vi "VRM.Get Target.vi"(6 "Axis":T1=enum."Z", 8 "error in (no error)":errorcluster, 11 "Instrument.VRM in":refnum<class "Instrument.OxfordVRM.lvclass">) -> (0 "error out":errorcluster, 1 "Target Field Rate (T/min)":dbl[](array[numeric]), 2 "Target Field (T)":dbl[](array[numeric]), 3 "Instrument.VRM out":refnum<class "Instrument.OxfordVRM.lvclass">)   [LabVIEW 2019, in "Instrument.OxfordVRM.lvclass"]
uses:
  Instrument.OxfordVRM.lvclass
  Typedefs/VRM Magnet Axis--Enum.ctl
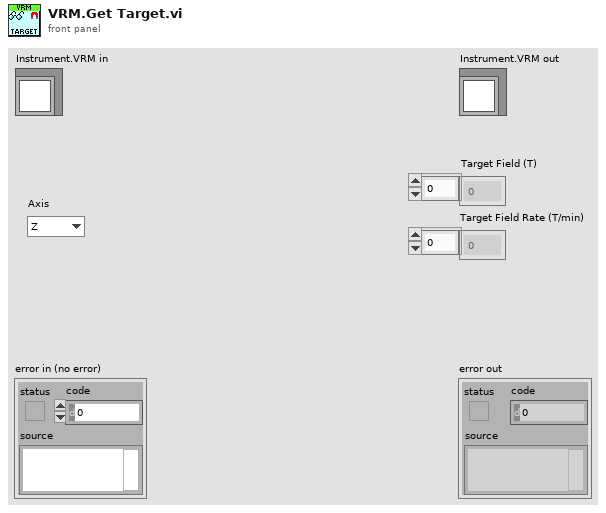
[diagram p1: front panel]
types:
  T1 = typedef "Instrument.OxfordVRM.lvclass/VRM Magnet Axis--Enum.ctl" = enum16{"X", "Y", "Z", "ALL"}
  T2 = typedef "Instrument.Cryostat.lvclass/Magnet Axis--Enum.ctl" = enum16{"X", "Y", "Z"}
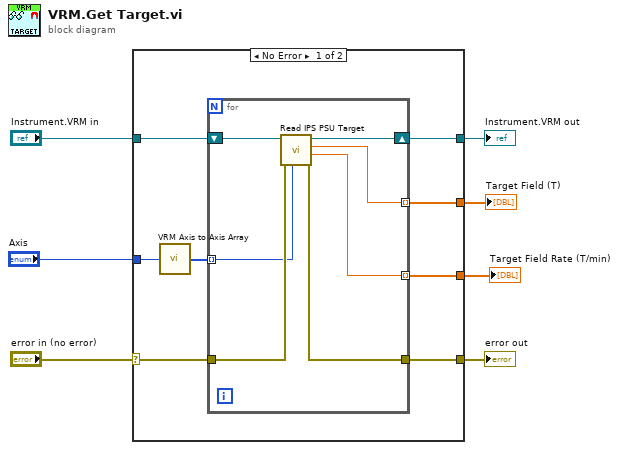
[diagram p0: block diagram]
diagram:
  n1 = case shown="No Error" "error in (no error)" {
    selector: "error in (no error)" -> [w13 w24]
    tunnel: [w12 w24] -> w6
    tunnel: [w14 w23] -> w4
    tunnel: "Instrument.VRM in" -> [w15 w23]
    tunnel: [w9 _] -> w1
    tunnel: "Axis" -> [w11 _]
    tunnel: [w10 _] -> w2
    frame No Error {
      n2 = call "VRM Axis to Axis Array.vi"("Axis"=w11) -> ("Axis Array"=w8:T2[])
      n3 = for {
        tunnel: w8 -> [w17] mode=indexing
        tunnel: [w20] -> w10 mode=indexing
        tunnel: [w19] -> w9 mode=indexing
        shift-right: [w21] -> w14
        shift-left: w15 -> [w22]
        tunnel: w13 -> [w18]
        tunnel: [w16] -> w12
        n4 = call "Read IPS PSU Target.vi"("Axis"=w17, "error in (no error)"=w18, "Instrument.OxfordVRM in"=w22) -> ("error out"=w16:errorcluster, "Target Field Rate (T/min)"=w20:dbl, "Target Field (T)"=w19:dbl, "Instrument.OxfordVRM out"=w21:refnum<class "Instrument.OxfordVRM.lvclass">)  [unwired: 5 in]
      }
    }
    frame Error {
    }
  }
  "error out" <- w6
  "Instrument.VRM out" <- w4
  "Target Field (T)" <- w1
  "Target Field Rate (T/min)" <- w2
